vi "Download Waveforms.vi"(0 "fpga interface in":refnum<k20>, 5 "stream instance":u32, 7 "waveforms":waveform(dbl)[](array[waveform]), 11 "error in":errorcluster) -> (4 "fpga interface out":refnum<k20>, 6 "stream instance out":u32, 15 "error out":errorcluster)   [LabVIEW 2018, in "GettingStarted_5785_Host.lvlib"]
uses:
  GettingStarted_5785_Host.lvlib
  <instrlib>/FlexRIO/API/Host/v1/NI FlexRIO/API/Get Property Reference - Fpga Small.vi
  <resource>/objmgr/niflexrioapiChannel.rc
  <instrlib>/FlexRIO/API/Host/v1/NI FlexRIO API v1.lvlib
  <resource>/objmgr/niflexrioapiStream.rc
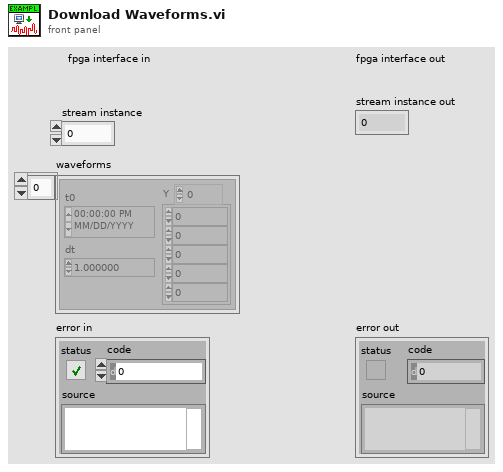
[diagram p1: front panel]
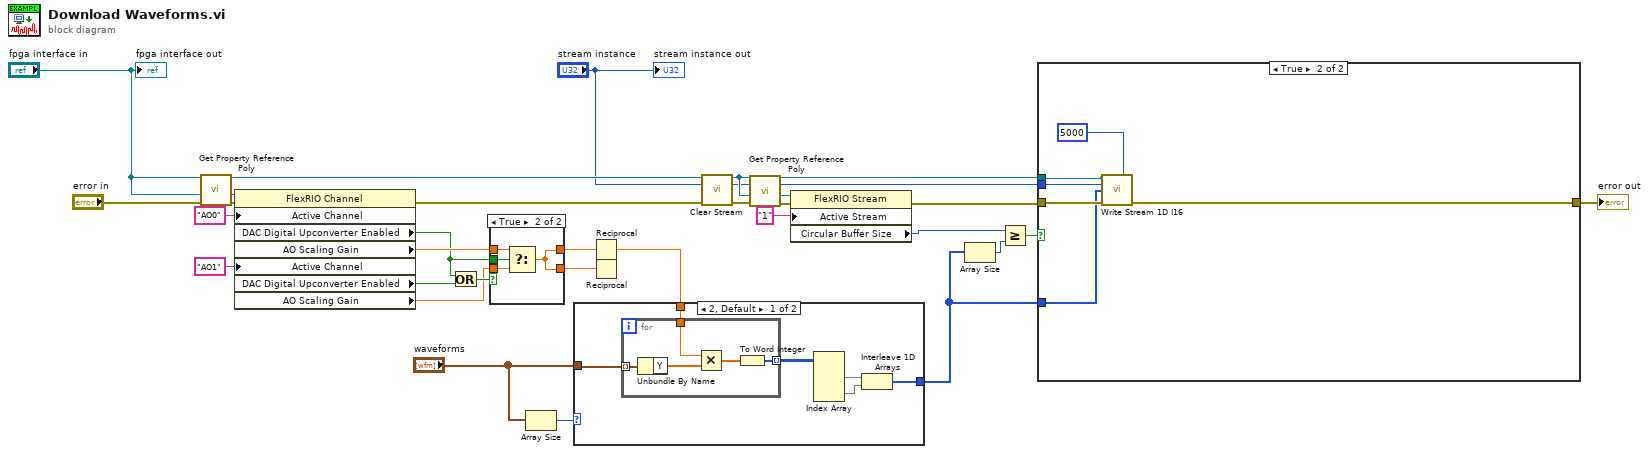
[diagram p0: block diagram]
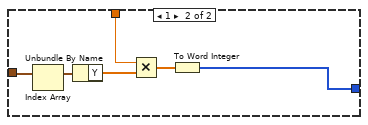
[diagram p2: hidden frame]
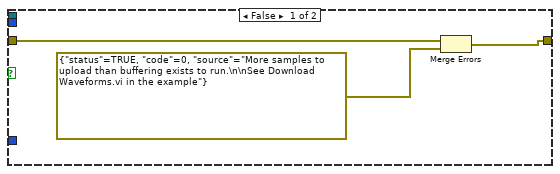
[diagram p4: hidden frame]
diagram:
  n1 = call-poly <instrlib>:"Get Property Reference Poly.vi"("error in (no error)"="error in", "fpga interface in"="fpga interface in") -> ("error out"=w17:errorcluster, "property reference"=w16:refnum<k20>)  [unwired: 4 in, 1 out]
  n2 = property class="FlexRIO Channel"(reference=w16, error in=w17, "Active Channel"="AO0", "Active Channel"="AO1") -> (error out=w13:errorcluster, "DAC Digital Upconverter Enabled"=w20:bool, "AO Scaling Gain"=w22:dbl, "DAC Digital Upconverter Enabled"=w23:bool, "AO Scaling Gain"=w21:dbl)  [unwired: 1 out]
  n3 = Or(x=w20, y=w23) -> (x .or. y?=w24:bool)
  n4 = case shown="True" w24 {
    tunnel: w22 -> [w32 w35]
    tunnel: w21 -> [w31 w34]
    tunnel: [w32 w33] -> w18
    tunnel: [w31 w33] -> w19
    tunnel: w20 -> [_ w36]
    frame False {
    }
    frame True {
      n5 = Select(t=w35, s=w36, f=w34) -> (s? t:f=w33:dbl)
    }
  }
  n6 = Array Size(array="waveforms") -> (size(s)=w9:i32)
  n7 = Reciprocal(x=w18) -> (1/x=w12:dbl)
  n8 = case shown="2, Default" w9 {
    tunnel: w12 -> [w42 w53]
    tunnel: [w38 w48] -> w11
    tunnel: "waveforms" -> [w37 w52]
    frame 2, Default {
      n9 = for {
        tunnel: w37 -> [w47] mode=indexing
        tunnel: w42 -> [w45]
        tunnel: [w43] -> w41 mode=indexing
        n10 = Unbundle By Name(w47) -> ("Y"=w46:dbl[])
        n11 = Multiply(x=w45, y=w46) -> (x*y=w44:dbl[])
        n12 = To Word Integer(number=w44) -> (16bit integer=w43:i16[])
      }
      n13 = Index Array(array=w41) -> (element #1=w40:i16[], element #2=w39:i16[])  [unwired: 4 in]
      n14 = Interleave 1D Arrays(w40, w39) -> (w38:i16[])
    }
    frame 1 {
      n15 = Index Array(array=w52) -> (element=w49:waveform(dbl))  [unwired: 1 in]
      n16 = Unbundle By Name(w49) -> ("Y"=w51:dbl[])
      n17 = Multiply(x=w53, y=w51) -> (x*y=w50:dbl[])
      n18 = To Word Integer(number=w50) -> (16bit integer=w48:i16[])
    }
  }
  n19 = Reciprocal(x=w19) -> ()  [unwired: 1 out]
  n20 = call <instrlib>:"Clear Stream.vi"("fpga interface in"="fpga interface in", "stream instance"="stream instance", "error in"=w13) -> ("fpga interface out"=w3:refnum<k20>, "stream instance out"=w1:u32, "error out"=w4:errorcluster)  [unwired: 10 in]
  n21 = call-poly <instrlib>:"Get Property Reference Poly.vi"("error in (no error)"=w4, "fpga interface in"=w3) -> ("error out"=w8:errorcluster, "property reference"=w7:refnum<k20>)  [unwired: 4 in, 1 out]
  n22 = property class="FlexRIO Stream"(reference=w7, error in=w8, "Active Stream"="1") -> (error out=w2:errorcluster, "Circular Buffer Size"=w5:u64)  [unwired: 1 out]
  n23 = Array Size(array=w11) -> (size(s)=w27:i32)
  n24 = Greater Or Equal?(x=w5, y=w27) -> (x >= y?=w28:bool)
  n25 = case shown="True" w28 {
    tunnel: w3 -> [_ w61]
    tunnel: w2 -> [w56 w62]
    tunnel: w11 -> [_ w59]
    tunnel: [w54 w58] -> w29
    tunnel: w1 -> [_ w60]
    frame False {
      n26 = Merge Errors(w56, errorcluster {"status"=TRUE, "code"=0, "source"="More samples to upload than buffering exists to run.\n\nSee Download Waveforms.vi in the example"} ("error in")) -> (w54:errorcluster)
    }
    frame True {
      n27 = call <instrlib>:"Write Stream 1D I16.vi"("fpga interface in"=w61, "timeout"=5000, "stream instance"=w60, "write data"=w59, "error in"=w62) -> ("error out"=w58:errorcluster)  [unwired: 8 in, 2 out]
    }
  }
  "error out" <- w29
  "fpga interface out" <- "fpga interface in"
  "stream instance out" <- "stream instance"
